vi "String(Float with Unit) To Float Example.vi"() -> ()   [LabVIEW 2017]
uses:
  API-String-Arugments-Support/API String Arguments Support.lvlib
panel:
  out "Array":T1(array[cluster])
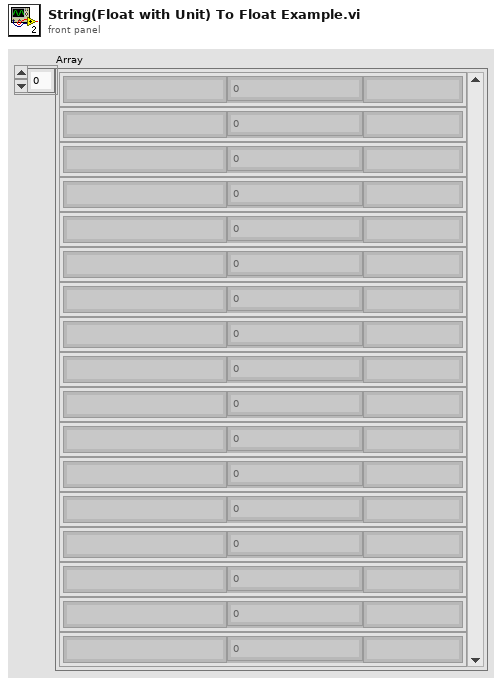
[diagram p1: front panel]
types:
  T1 = cluster{"String":string, "Float":dbl, "Unit String":string}[]
  T2 = cluster{"String":string, "Float":dbl, "Unit String":string}
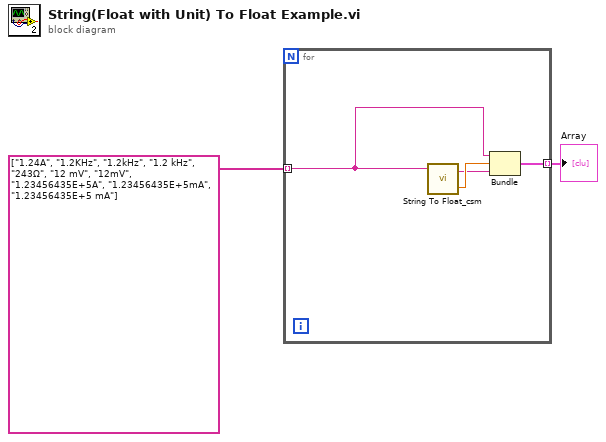
[diagram p0: block diagram]
diagram:
  n1 = for {
    tunnel: string[] ["1.24A", "1.2KHz", "1.2kHz", "1.2 kHz", "243Ω", "12 mV", "12mV", "1.23456435E+5A", "1.23456435E+5mA", "1.23456435E+5 mA"] ("String") -> [w5] mode=indexing
    tunnel: [w6] -> w1 mode=indexing
    n2 = call "String To Float_csm.vi"("String"=w5) -> ("Float"=w4:dbl, "Unit String"=w3:string)  [unwired: 3 in]
    n3 = Bundle("String"=w5, "Float"=w4, "Unit String"=w3) -> (w6:T2)  [unwired: 1 in]
  }
  "Array" <- w1
